vi "SCT Decode Type Descriptor.vi"(8 "error in (no error)":errorcluster, 11 "Encoded Type":string) -> (0 "error out":errorcluster, 3 "Type Descriptor":T1)   [LabVIEW 2016]
uses:
  <vilib>/variable/Type Descriptor.ctl
  <vilib>/variable/NI_Variable.lvlib
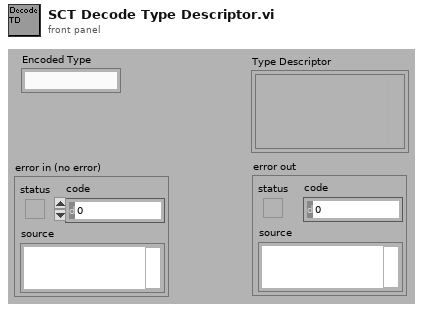
[diagram p1: front panel]
types:
  T1 = typedef "NI_Variable.lvlib/Type Descriptor.ctl" = cluster{"Variant":variant}
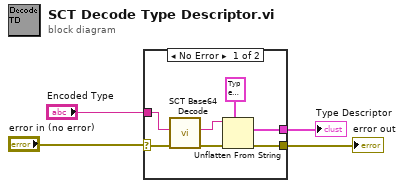
[diagram p0: block diagram]
diagram:
  n1 = case shown="No Error" "error in (no error)" {
    selector: "error in (no error)" -> [w6 w12]
    tunnel: "Encoded Type" -> [w11 _]
    tunnel: [w8 _] -> w3
    tunnel: [w7 w12] -> w1
    frame No Error {
      n2 = call <resource>:"SCT Base64 Decode.vi"("error in (no error)"=w6, "buffer in"=w11) -> ("error out"=w5:errorcluster, "base64 decoded buffer"=w10:string)  [unwired: 8 in]
      n3 = Unflatten From String(type=T1 {"Variant"=variant} ("Type Descriptor"), binary string=w10, error in (no error)=w5) -> (value=w8:T1, error out=w7:errorcluster)  [unwired: 2 in, 1 out]
    }
    frame Error {
    }
  }
  "Type Descriptor" <- w3
  "error out" <- w1
